vi "@create.vi"(6 "autorun? (false)":bool, 7 "dotnet_system_exec in":refnum<class "dotnet_system_exec.lvclass">, 8 "error in (no error)":errorcluster, 9 "working directory (c:\\)":path=path "c:/", 10 "arguments (\"\")":string, 11 "command line (cmd.exe)":string="cmd.exe") -> (0 "error out":errorcluster, 2 "public events":T1, 3 "dotnet_system_exec out":refnum<class "dotnet_system_exec.lvclass">)   [LabVIEW 2013, in "dotnet_system_exec.lvclass"]
doc: "Creates an instance of the .NET System Process. It configures the instance not to show a window but to redirect the stdout, stderr, and stdin so that LabVIEW can interface with them. Use the public events to register for the stdout and stderr events."
uses:
  dotnet_system_exec.lvclass
  dotnet_system_exec.lvclass/dotnet_system_exec.ctl
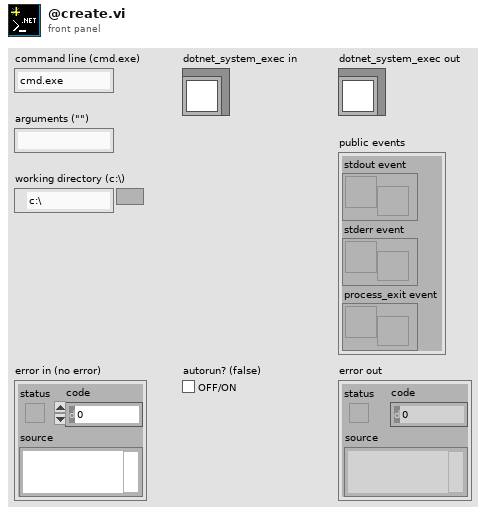
[diagram p1: front panel]
types:
  T1 = cluster{"stdout event":refnum<user-event>, "stderr event":refnum<user-event>, "process_exit event":refnum<user-event>}
  T2 = cluster{"StdOut Event":refnum<user-event>, "StdErr Event":refnum<user-event>, "ProcessExit Event":refnum<user-event>}
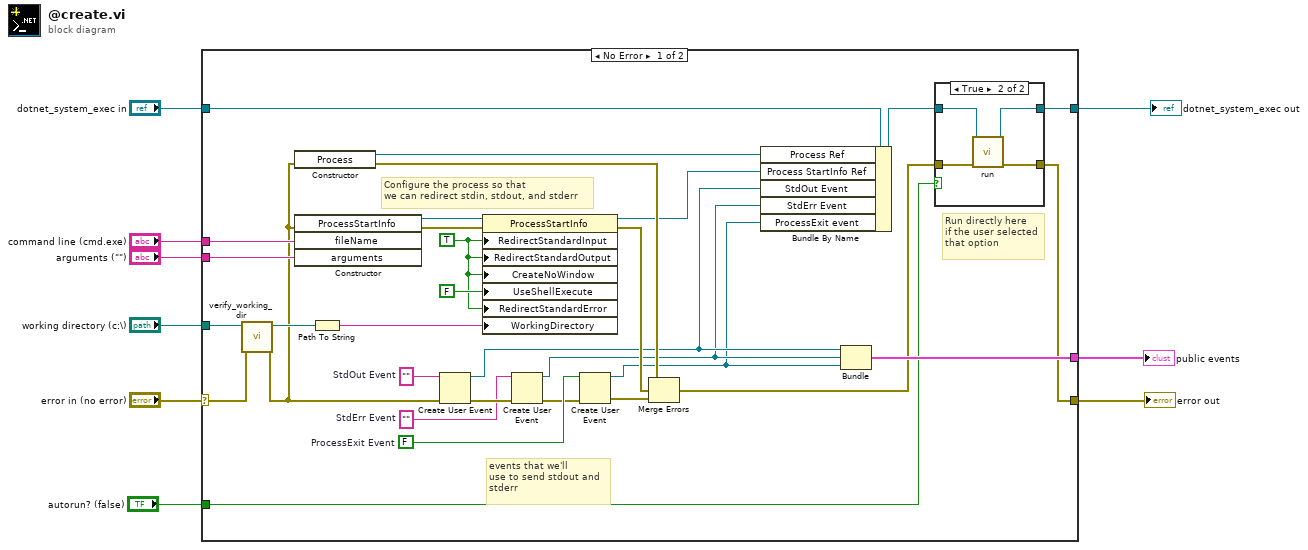
[diagram p0: block diagram]
diagram:
  n1 = case shown="No Error" "error in (no error)" {
    selector: "error in (no error)" -> [w11 w48]
    tunnel: [w19 w48] -> w8
    tunnel: [w21 w47] -> w6
    tunnel: "dotnet_system_exec in" -> [w31 w47]
    tunnel: "command line (cmd.exe)" -> [w34 _]
    tunnel: "arguments (\"\")" -> [w33 _]
    tunnel: "working directory (c:\\)" -> [w13 _]
    tunnel: [w25 _] -> w3
    tunnel: "autorun? (false)" -> [w18 _]
    frame No Error {
      w17 = FALSE  # ProcessExit Event
      w26 = ""  # StdErr Event
      w28 = ""  # StdOut Event
      w37 = TRUE ("RedirectStandardInput")
      # "Configure the process so that\nwe can redirect stdin, stdout, and stderr"
      # "events that we'll\nuse to send stdout and\nstderr"
      # "Run directly here\nif the user selected\nthat option"
      n2 = call "verify_working_dir.vi"("error in (no error)"=w11, "working directory"=w13) -> ("error out"=w10:errorcluster, "working directory out"=w12:path)  [unwired: 8 in]
      n3 = constructor class="Process"(error in=w10) -> (reference out=w30:refnum<k24>, error out=w36:errorcluster)  [unwired: 2 in, 1 out]
      n4 = constructor class="ProcessStartInfo"(error in=w10, "fileName"=w34, "arguments"=w33) -> (reference out=w39:refnum<k24>, error out=w40:errorcluster)  [unwired: 2 in, 3 out]
      n5 = Path To String(path=w12) -> (string=w32:string)
      n6 = Create User Event(user event datatype=w28, error in=w10) -> (user event=w24:refnum<user-event>, error out=w27:errorcluster)
      n7 = property class="ProcessStartInfo"(reference=w39, error in=w40, "RedirectStandardInput"=w37, "RedirectStandardOutput"=w37, "CreateNoWindow"=w37, "UseShellExecute"=FALSE, "RedirectStandardError"=w37, "WorkingDirectory"=w32) -> (reference out=w29:refnum<k24>, error out=w35:errorcluster)
      n8 = Create User Event(user event datatype=w26, error in=w27) -> (user event=w23:refnum<user-event>, error out=w16:errorcluster)
      n9 = Create User Event(user event datatype=w17, error in=w16) -> (user event=w14:refnum<user-event>, error out=w15:errorcluster)
      n10 = Merge Errors(w36, w35, w15) -> (w20:errorcluster)
      n11 = Bundle By Name(cluster=w31, "Process Ref"=w30, "Process StartInfo Ref"=w29, "StdOut Event"=w24, "StdErr Event"=w23, "ProcessExit event"=w14) -> (w22:refnum<class "dotnet_system_exec.lvclass">)
      n12 = Bundle("StdOut Event"=w24, "StdErr Event"=w23, "ProcessExit Event"=w14) -> (w25:T2)  [unwired: 1 in]
      n13 = case shown="True" w18 {
        tunnel: w22 -> [w42 w46]
        tunnel: [w42 w45] -> w21
        tunnel: w20 -> [w41 w44]
        tunnel: [w41 w43] -> w19
        frame False {
        }
        frame True {
          n14 = call "run.vi"("error in (no error)"=w44, "dotnet_system_exec in"=w46) -> ("error out"=w43:errorcluster, "dotnet_system_exec out"=w45:refnum<class "dotnet_system_exec.lvclass">)  [unwired: 8 in]
        }
      }
    }
    frame Error {
    }
  }
  "error out" <- w8
  "dotnet_system_exec out" <- w6
  "public events" <- w3
